vi "Get Version String.vi"(8 "error in (no error)":errorcluster) -> (0 "error out":errorcluster, 3 "version info string":string)   [LabVIEW 2020, in "Get COM Descriptor.lvlib"]
doc: "Get DLL version string."
uses:
  Get COM Descriptor.lvlib
  get_com_descriptor.dll
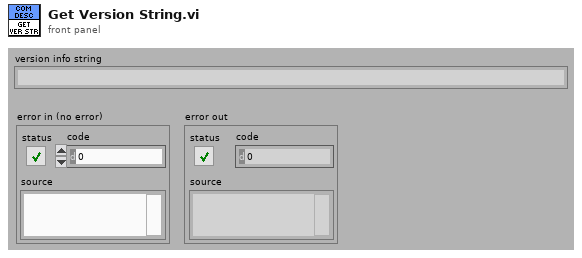
[diagram p1: front panel]
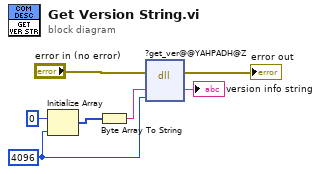
[diagram p0: block diagram]
diagram:
  w2 = 4096 ("dimension size")
  n1 = Initialize Array(u8 0 ("element"), w2) -> (w5:u8[])
  n2 = Byte Array To String(unsigned byte array=w5) -> (string=w3:string)
  n3 = dll-call lib="F:/z-bridge-v4/other/get_com_descriptor/get_com_descriptor.dll" fn="?get_ver@@YAHPADH@Z"(error in="error in (no error)", "buf"=w3, "size"=w2) -> (error out=→"error out":errorcluster, "buf"=→"version info string":string)  [unwired: 4 in, 1 out]
